vi "DAQmx Create Channel (AI-Torque-Bridge-Polynomial).vi"(0 "task in":refnum<k21>, 1 "maximum value":dbl=100.0 format="%0.2f", 2 "minimum value":dbl=-100.0 format="%0.2f", 3 "bridge information":T1={"bridge configuration"=10182, "voltage excitation source"=10200, "voltage excitation value"=2.5, "nominal bridge resistance"=350.0} {"voltage excitation source" items=["Internal"=10200, "External"=10167]; "bridge configuration" items=["Full Bridge"=10182, "Half Bridge"=10187, "Quarter Bridge"=10270]}, 5 "physical channels":tag, 7 "name to assign":string, 9 "units":i32(ring)=15883 items=["Nm"=15881, "oz-in"=15882, "lb-in"=15883, "lb-ft"=15884, "From Custom Scale"=10065], 11 "error in":errorcluster, 12 "custom scale name":tag, 14 "scaling information":T2={"forward coeff"=[0.0, 50.0], "reverse coeff"=[0.0, 0.02], "electrical units"=15897, "physical units"=15883} {"electrical units" items=["Volts/Volt"=15896, "mVolts/Volt"=15897]; "physical units" items=["Nm"=15881, "oz-in"=15882, "lb-in"=15883, "lb-ft"=15884]}) -> (4 "task out":refnum<k21>, 15 "error out":errorcluster)   [LabVIEW 2024]
doc: "Creates channel(s) that use a Wheatstone bridge to measure torque. Use this instance with sensors whose specifications provide a polynomial to convert electrical values to physical values. When you use this scaling type, NI-DAQmx requires coefficients for a polynomial that converts electrical values to physical values (forward), as well as coefficients for a polynomial that converts physical values to electrical values (reverse). If you only know one set of coefficients, use the DAQmx Compute Reverse Polynomial Coefficients VI to generate the other set."
uses:
  nilvaiu.dll
panel:
  # "input limits"
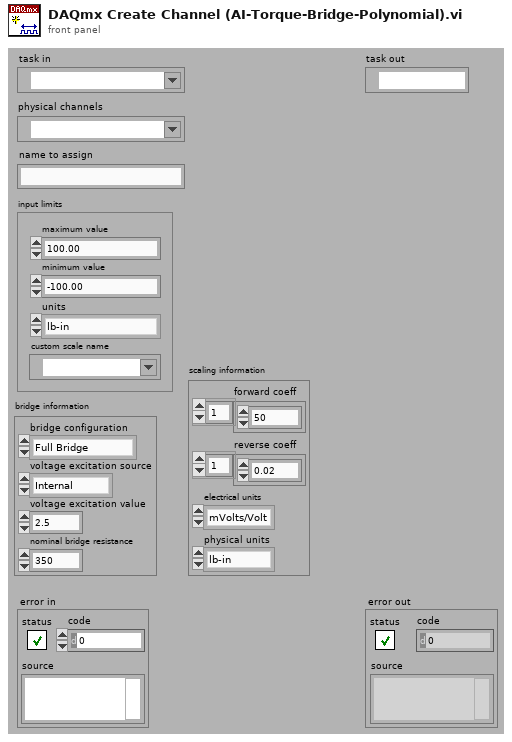
[diagram p1: front panel]
types:
  T1 = cluster{"bridge configuration":i32, "voltage excitation source":i32, "voltage excitation value":dbl, "nominal bridge resistance":dbl}
  T2 = cluster{"forward coeff":dbl[], "reverse coeff":dbl[], "electrical units":i32, "physical units":i32}
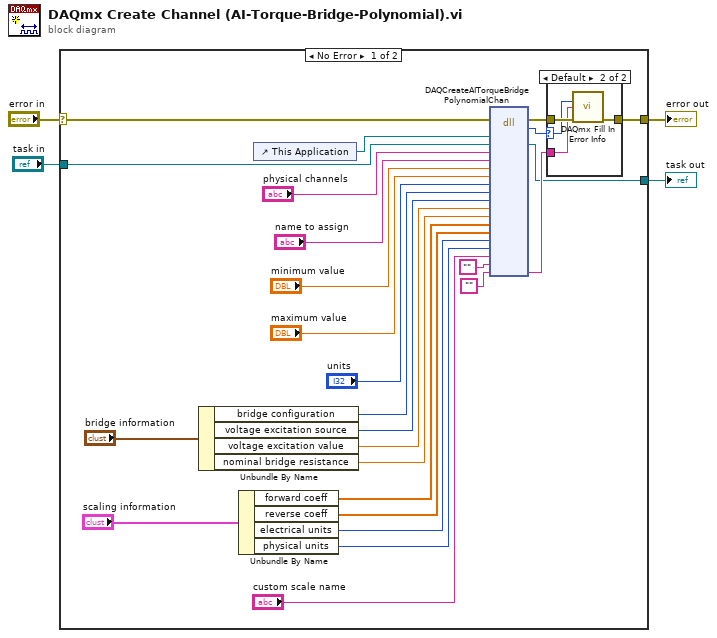
[diagram p0: block diagram]
diagram:
  n1 = case shown="No Error" "error in" {
    selector: "error in" -> [w8 w36]
    tunnel: "task in" -> [w10 w37]
    tunnel: [w9 w37] -> w3
    tunnel: [w7 w36] -> w1
    frame No Error {
      n2 = Unbundle By Name("bridge information") -> ("bridge configuration"=w20:i32, "voltage excitation source"=w21:i32, "voltage excitation value"=w22:dbl, "nominal bridge resistance"=w29:dbl)
      n3 = Unbundle By Name("scaling information") -> ("forward coeff"=w16:dbl[], "reverse coeff"=w17:dbl[], "electrical units"=w18:i32, "physical units"=w19:i32)
      n4 = control-ref of="This Application"() -> (w28:refnum<vi>)
      n5 = dll-call lib="nilvaiu.*" fn="DAQCreateAITorqueBridgePolynomialChan"(error in=w8, "lvAppRef"=w28, "refObjPtr"=w10, "physicalChannelName"="physical channels", "channelNameIn"="name to assign", "minVal"="minimum value", "maxVal"="maximum value", "units"="units", "bridgeConfig"=w20, "voltageExcitSource"=w21, "voltageExcitVal"=w22, "nominalBridgeResistance"=w29, "forwardCoeffs"=w16, "reverseCoeffs"=w17, "electricalUnits"=w18, "physicalUnits"=w19, "customScaleName"="custom scale name", "channelNamesOut"="", "extendedErrorInfo"="") -> (error out=w30:errorcluster, "return type"=w26:i32, "refObjPtr"=w9:refnum<k21>, "extendedErrorInfo"=w27:string)  [unwired: 18 in, 1 out]
      n6 = case shown="Default" w26 {
        selector: w26 -> [_ w33]
        tunnel: w30 -> [w31 w35]
        tunnel: [w31 w34] -> w7
        tunnel: w27 -> [_ w32]
        frame 0 {
        }
        frame Default {
          n7 = call "DAQmx Fill In Error Info.vi"("status code"=w33, "extended error info"=w32, "error in"=w35) -> ("error out"=w34:errorcluster)  [unwired: 1 in, 11 out]
        }
      }
    }
    frame Error {
    }
  }
  "task out" <- w3
  "error out" <- w1
